vi "usrp tx (2).vi"() -> ()   [LabVIEW 2014]
uses:
  <instrlib>/niUSRP/niUSRP Write Tx Data (CDB).vi
  <vilib>/measure/NI_MABase.lvlib
panel:
  in  "duty cycle (%)":dbl=50.0 format="%0.2f"
  in  "stop":bool
  in  "sampling info":cluster{"Fs":dbl, "#s":dbl}={"Fs"=1000.0, "#s"=1000.0} {"Fs" format="%.2p"}
  in  "active antenna":string
  in  "gain":dbl format="%#_6f"
  in  "channel list":string
  in  "frequency":dbl=10.0 format="%0.2p"
  out "Waveform Graph":waveform(dbl)(graph)
  in  "signal type":T1(ring)
  in  "carrier frequency":dbl=100000.0 format="%#_6p"
  in  "IQ rate":dbl=100000.0 format="%#_6p"
  in  "device names":refnum<k15>
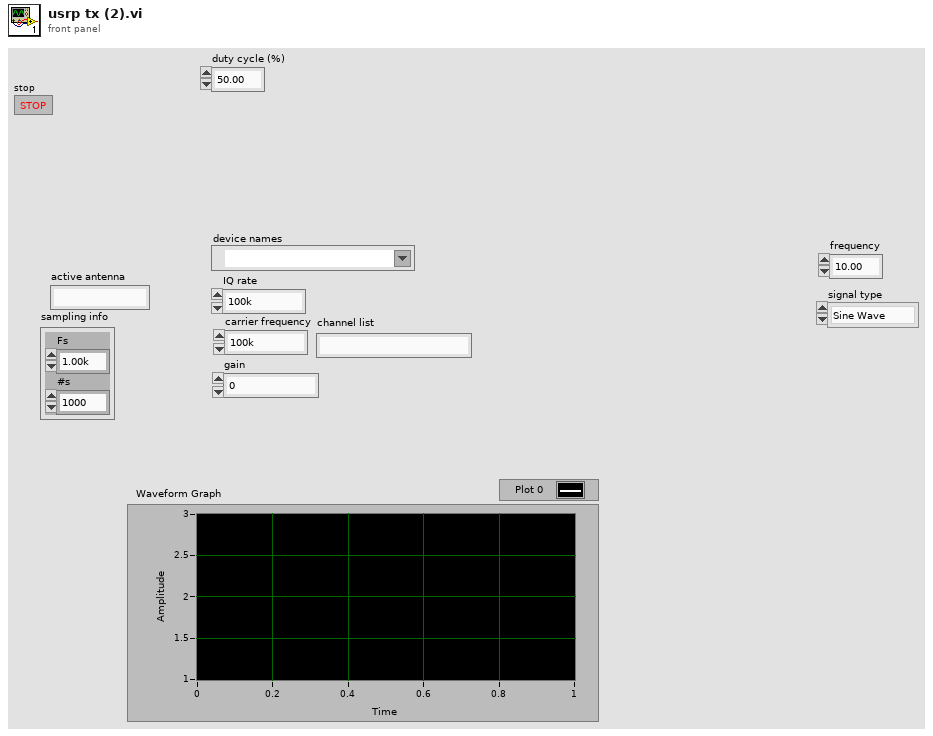
[diagram p1: front panel]
types:
  T1 = enum16{"Sine Wave", "Triangle Wave", "Square Wave", "Sawtooth Wave"}
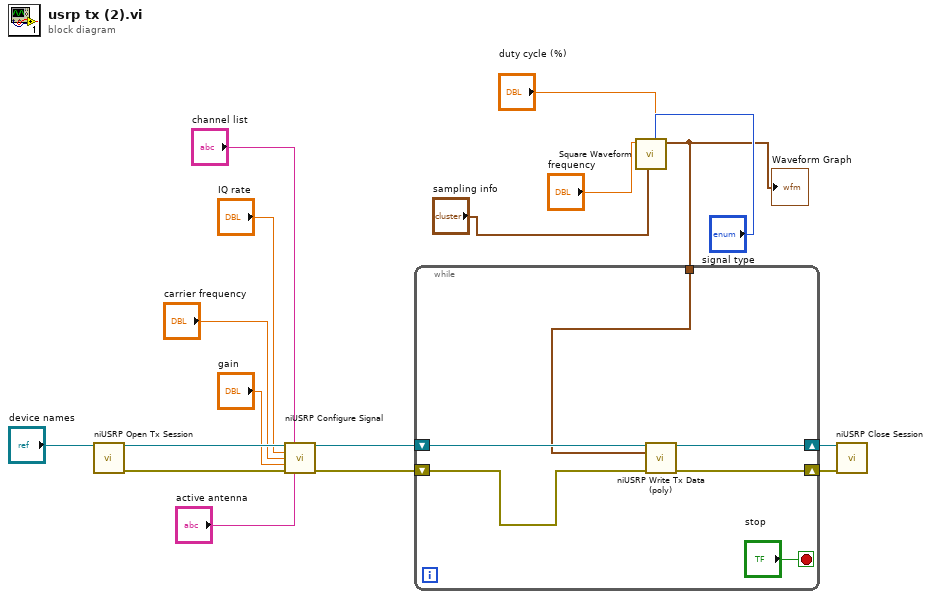
[diagram p0: block diagram]
diagram:
  n1 = call <instrlib>:"niUSRP Open Tx Session.vi"("device names"="device names") -> ("session handle out"=w16:refnum<k15>, "error out"=w15:errorcluster)  [unwired: 13 in]
  n2 = call <instrlib>:"niUSRP Configure Signal.vi"("session handle"=w16, "channel list"="channel list", "IQ rate"="IQ rate", "carrier frequency"="carrier frequency", "gain"="gain", "error in (no error)"=w15, "active antenna"="active antenna") -> ("session handle out"=w14:refnum<k15>, "error out"=w13:errorcluster)  [unwired: 4 in, 3 out]
  n3 = call <vilib>:"Square Waveform.vi"("duty cycle (%)"="duty cycle (%)", "offset"="signal type", "sampling info"="sampling info", "frequency"="frequency") -> ("signal out"=w2:waveform(dbl))  [unwired: 6 in, 1 out]
  "Waveform Graph" <- w2
  n4 = while {
    shift-right: [w23] -> w12
    shift-left: w14 -> [w21]
    shift-right: [w22] -> w11
    shift-left: w13 -> [w19]
    tunnel: w2 -> [w20]
    stop <- "stop" stop-if-true
    n5 = call-poly <instrlib>:"niUSRP Write Tx Data (poly).vi"("session handle"=w21, "data"=w20, "error in (no error)"=w19) -> ("session handle out"=w23:refnum<k15>, "error out"=w22:errorcluster)  [unwired: 11 in]
  }
  n6 = call <instrlib>:"niUSRP Close Session.vi"("session handle"=w12, "error in (no error)"=w11) -> ()  [unwired: 13 in, 1 out]
